vi "Close Local UDP Connection.vi"(8 "error in":errorcluster, 11 "Local UDP Connection ref":refnum<k16>) -> (0 "Error out":errorcluster)   [LabVIEW 2021, in "UDP Comms.lvlib"]
uses:
  UDP Comms.lvlib
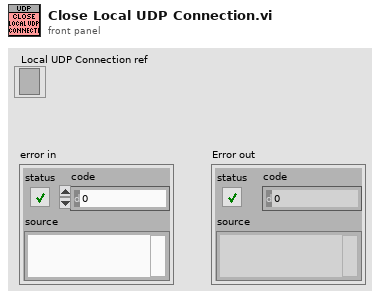
[diagram p1: front panel]
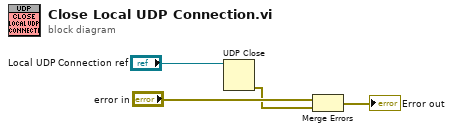
[diagram p0: block diagram]
diagram:
  n1 = UDP Close(connection ID="Local UDP Connection ref") -> (error out=w2:errorcluster)  [unwired: 1 in, 1 out]
  n2 = Merge Errors("error in", w2) -> (→"Error out":errorcluster)
